vi "Does the Checksum thing work.vi"() -> ()   [LabVIEW 2010]
panel:
  out "Boolean":bool
  out "CS string in 2":string
  in  "Data String In":string
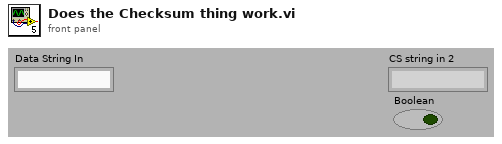
[diagram p1: front panel]
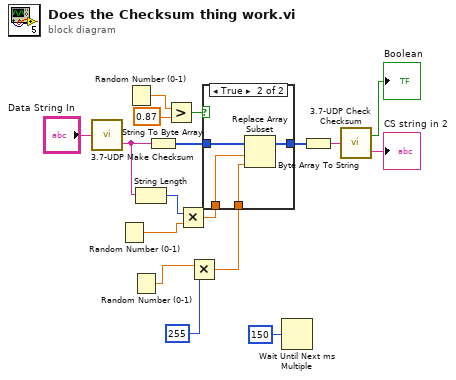
[diagram p0: block diagram]
diagram:
  n1 = call "3.7-UDP Make Checksum.vi"("Data String In"="Data String In") -> ("CS String Out"=w8:string)  [unwired: 1 out]
  n2 = Random Number (0-1)() -> (number: 0 to 1=w6:dbl)
  n3 = Random Number (0-1)() -> (number: 0 to 1=w11:dbl)
  n4 = Random Number (0-1)() -> (number: 0 to 1=w3:dbl)
  n5 = String Length(string=w8) -> (length=w7:i32)
  n6 = String To Byte Array(string=w8) -> (unsigned byte array=w14:u8[])
  n7 = Greater?(x=w11, y=0.87) -> (0:w9:bool)
  n8 = Multiply(x=w7, y=w6) -> (x*y=w5:dbl)
  n9 = Multiply(x=w3, y=255) -> (x*y=w2:dbl)
  n10 = case shown="True" w9 {
    tunnel: w14 -> [w18 w22]
    tunnel: [w18 w21] -> w12
    tunnel: w5 -> [_ w20]
    tunnel: w2 -> [_ w19]
    frame False {
    }
    frame True {
      n11 = Replace Array Subset(array=w22, new element=w19, index=w20) -> (w21:u8[])
    }
  }
  n12 = Wait Until Next ms Multiple(millisecond multiple=u32 150) -> ()  [unwired: 1 out]
  n13 = Byte Array To String(unsigned byte array=w12) -> (string=w13:string)
  n14 = call "3.7-UDP Check Checksum.vi"("CS string in"=w13) -> ("CS string in 2"=→"CS string in 2":string, "Boolean"=→"Boolean":bool)
